vi "Load Settings.vi"(8 "error in (no error)":errorcluster {"code" format="Error %.0f"}, 11 "Printer Settings In":refnum<class "Printer Settings.lvclass">) -> (0 "error out":errorcluster {"code" format="Error %.0f"}, 3 "Printer Settings Out":refnum<class "Printer Settings.lvclass">)   [LabVIEW 2023, in "VIDoc Printer.lvlib" / "Printer Settings.lvclass"]
uses:
  Printer Settings.lvclass
  C:/projects/DMC/Tooling/Git-Action-Service/Source/Documentation Generation/Settings/VIDoc Settings/VIDoc Settings.lvclass
  VIDoc Settings/VIDoc Settings.lvclass/VIDoc Settings.ctl
  Printer Settings.lvclass/Printer Settings.ctl
  VIDoc Settings/Get VIDoc Settings Path.vi
  Parser Settings/Parser Settings.lvclass
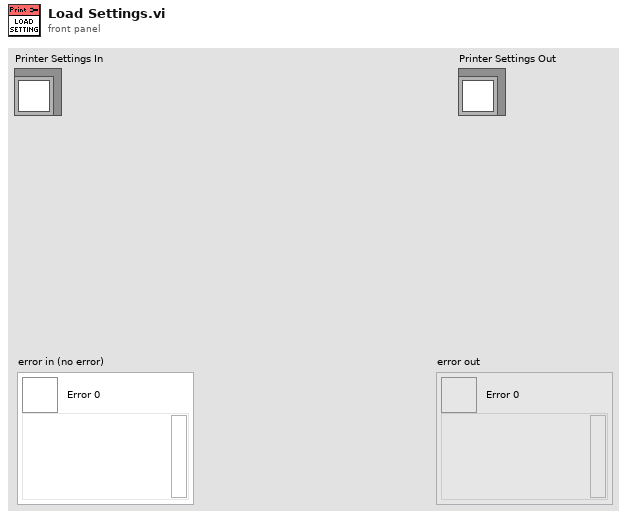
[diagram p1: front panel]
types:
  T1 = typedef "VIDoc Printer.lvlib/Printer Settings.lvclass/Enabled Sections Cluster.ctl" = cluster{"Projects":bool, "Interfaces":bool, "Classes":bool, "Libraries":bool, "VIs":bool, "Controls":bool, "LLBs":bool}
  T2 = typedef "VIDoc Printer.lvlib/Printer Settings.lvclass/Printer Settings Cluster.ctl" = cluster{"Project":T3, "VI Member":T4, "Interface":T6, "Class":T8, "Library":T9, "Control Member":T10, "Format Options":T11, "Library Scope":cluster{"Public":bool, "Community":bool, "Private":bool, "Unknown":bool}, "LLB":T14, "Bookmark Settings Map":map{string, T4}}
  T3 = typedef "VIDoc Printer.lvlib/Printer Settings.lvclass/Project Settings.ctl" = cluster{"Paths":bool, "Descriptions":bool, "Memory":bool, "Options":bool, "Symbols":bool}
  T4 = typedef "VIDoc Printer.lvlib/Printer Settings.lvclass/VI Settings.ctl" = cluster{"Memory":bool, "By Folder":bool, "By Tree":bool, "By List":bool, "Methods":bool, "Method Options":cluster{"Front Panels":bool, "Options":bool, "Controls":bool}, "List Detail Level":T5, "Methods Detail Level":T5, "Controls Detail Level":T5}
  T5 = typedef "VIDoc Printer.lvlib/Printer Settings.lvclass/Detail Level Enum.ctl" = enum16{"None", "Minimal", "Standard", "Full"}
  T6 = typedef "VIDoc Printer.lvlib/Printer Settings.lvclass/Interface Settings.ctl" = cluster{"Memory":bool, "By List":bool, "Details":bool, "Detail Options":cluster{"Description":bool, "Properties":bool, "Inheritance":bool, "Inheritance Options":cluster{"Parent Interfaces":bool, "Friends":bool}}, "List Detail Level":T5, "Controls Detail Level":T5, "Methods Detail Level":T5, "Controls Scope":T7, "Methods Scope":T7}
  T7 = typedef "VIDoc Printer.lvlib/Printer Settings.lvclass/Scope Settings.ctl" = cluster{"Public":bool, "Protected":bool, "Community":bool, "Private":bool, "Unknown":bool}
  T8 = typedef "VIDoc Printer.lvlib/Printer Settings.lvclass/Class Settings.ctl" = cluster{"Memory":bool, "By Folder":bool, "By Tree":bool, "By List":bool, "Details":bool, "Detail Options":cluster{"Description":bool, "Properties":bool, "Inheritance":bool, "Inheritance Options":cluster{"Parent Classes":bool, "Parent Interfaces":bool, "Parent Libraries":bool, "Friends":bool}}, "CPD Detail Level":T5, "List Detail Level":T5, "Controls Detail Level":T5, "Methods Detail Level":T5, "Set Accessor Detail Level":T5, "Get Accessor Detail Level":T5, "Controls Scope":T7, "Methods Scope":T7, "Get Accessors Scope":T7, "Set Accessors Scope":T7}
  T9 = typedef "VIDoc Printer.lvlib/Printer Settings.lvclass/Library Settings.ctl" = cluster{"Memory":bool, "By Folder":bool, "By Tree":bool, "By List":bool, "Details":bool, "Detail Options":cluster{"Description":bool, "Properties":bool, "Friends":bool, "Child Libraries":bool}, "List Detail Level":T5, "Methods Detail Level":T5, "Controls Detail Level":T5, "Methods Scope":T7, "Controls Scope":T7}
  T10 = typedef "VIDoc Printer.lvlib/Printer Settings.lvclass/Control Settings.ctl" = cluster{"Memory":bool, "By Folder":bool, "By Tree":bool, "By List":bool, "Controls":bool, "List Detail Level":T5, "Controls Detail Level":T5}
  T11 = typedef "VIDoc Printer.lvlib/Printer Settings.lvclass/Formatting Options.ctl" = cluster{"Background":cluster{"Public Scope":T12, "Protected Scope":T12, "Community Scope":T12, "Private Scope":T12, "Unknown Scope":T12, "Auto Error Handling":T12, "Inline":T12, "Separate CC":T12, "Execution Priority Normal":T12, "Reentrancy Non-RE":T12}, "Bookmark Options":T13}
  T12 = typedef "VIDoc Printer.lvlib/Printer Settings.lvclass/Background Formatting Cluster.ctl" = cluster{"Option":bool, "Color":u32, "Operator":bool}
  T13 = typedef "VIDoc Printer.lvlib/Printer Settings.lvclass/Bookmark Options.ctl" = cluster{"Bookmarks as New Line in VI Descriptions":bool, "Unique Bookmark Tags Only":bool, "Include Tag and Text":bool}
  T14 = typedef "VIDoc Printer.lvlib/Printer Settings.lvclass/LLB Settings.ctl" = cluster{"Methods":bool, "Controls":bool, "Methods Detail Level":T5, "Controls Detail Level":T5}
  T15 = typedef "VIDoc Parsing.lvlib/Parser Settings.lvclass/Parser Settings Cluster.ctl" = cluster{"Draw Controls":T16, "Max Control Recursion Depth":i32, "Bookmarks Map":map{string, string[]}}
  T16 = typedef "VIDoc Parsing.lvlib/Parser Settings.lvclass/Draw Controls Cluster.ctl" = cluster{"Subpanels":bool, "Tabs":bool, "TypeDefs":bool, "Error Clusters":T17, "DVRs":T17, "Queues & Notifiers":T17}
  T17 = typedef "VIDoc Parsing.lvlib/Parser Settings.lvclass/Draw Option Enum.ctl" = enum16{"Ignore", "Draw", "Draw + Contents"}
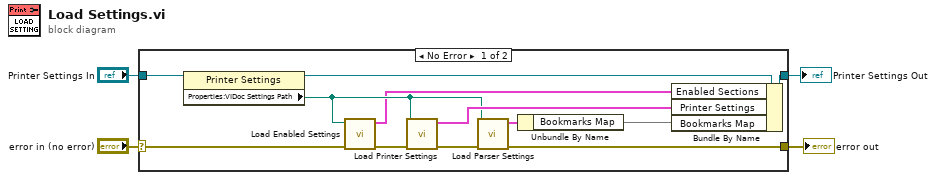
[diagram p0: block diagram]
diagram:
  n1 = case shown="No Error" "error in (no error)" {
    selector: "error in (no error)" -> [w13 w18]
    tunnel: [w9 w18] -> w2
    tunnel: [w14 w17] -> w1
    tunnel: "Printer Settings In" -> [w16 w17]
    frame No Error {
      n2 = property class="Printer Settings"(reference=w16) -> (reference out=w15:refnum<class "Printer Settings.lvclass">, "Properties:VIDoc Settings Path"=w8:path)  [unwired: 1 in, 1 out]
      n3 = call "Load Enabled Settings.vi"("Error in"=w13, "Settings Path"=w8) -> ("Error out"=w12:errorcluster, "Enabled Sections"=w7:T1)  [unwired: 7 in, 1 out]
      n4 = call "Load Printer Settings.vi"("Error in"=w12, "Settings Path"=w8) -> ("Error out"=w10:errorcluster, "Printer Settings"=w11:T2)  [unwired: 7 in, 1 out]
      n5 = call "Load Parser Settings.vi"("Error in"=w10, "Settings Path"=w8) -> ("Error out"=w9:errorcluster, "Parser Settings"=w6:T15)  [unwired: 7 in, 1 out]
      n6 = Unbundle By Name(w6) -> ("Bookmarks Map"=w5:map{string, string[]})
      n7 = Bundle By Name(cluster=w15, "Enabled Sections"=w7, "Printer Settings"=w11, "Bookmarks Map"=w5) -> (w14:refnum<class "Printer Settings.lvclass">)
    }
    frame Error {
    }
  }
  "error out" <- w2
  "Printer Settings Out" <- w1
